vi "JAUS Control Loop.vi"   [LabVIEW 2009]
uses:
  TypeDefs/State Machine/Main State.ctl
  <vilib>/Platform/TimedLoop/XDataNode/XDataNode.xnode
  <vilib>/Platform/TimedLoop/XDataNode/loadlvalarms.vi
  <vilib>/Platform/TimedLoop/XDataNode/timing_clust.ctl
  <vilib>/Platform/TimedLoop/XDataNode/nitl_modes.ctl
  <vilib>/Platform/TimedLoop/XDataNode/wakeup.ctl
  Functional Global Variables/Actions for FG's.ctl
  TypeDefs/Queue TypeDefs/Motor Instruction.ctl
  TypeDefs/Queue TypeDefs/Motor State.ctl
  Remote Control/Motor Command.ctl
  <vilib>/userDefined/High Color/nirio_resource_hc.ctl
  <vilib>/rvi/interface/nirviOpenFPGA/nirviOpenFPGA.xnode
  FPGA Bitfiles/Q_IGVC_2010.lvproj_FPGA Target_FPGA_MAIN.vi.lvbitx
  <vilib>/FPGAPlugInAG/cRIO-9113/nirviIntfOpen_cRIO-9113.vi
  <vilib>/Platform/TimedLoop/XDataNode/XDNodeRunTimeDep.lvlib
  <vilib>/NI_Real-Time Target Support.lvlib
  TypeDefs/Sensor TypeDefs/FPGA Main ref.ctl
types:
  T1 = typedef "Main State.ctl" = enum16{"Startup", "Wait for Init", "Initialize Sensors", "Wait for Saftey Disable", "Check Saftey", "Wait for GO", "Run", "Remote Control", "Stop"}
  T2 = typedef "XDNodeRunTimeDep.lvlib/timing_clust.ctl" = cluster{"Expected End [f-1]":u64, "Actual End [f-1]":u64, "Finished Late? [f-1]":bool, "Expected End [i-1]":u64, "Actual End [i-1]":u64, "Finished Late? [i-1]":bool, "Expected Start [i]":u64, "Actual Start [i]":u64, "Expected Start [f]":u64, "Actual Start [f]":u64, "Source Name":string, "Structure Name":string, "Period":i64, "Deadline":i64, "Offset":i64, "Start":i64, "Priority":i32, "Timeout":i32, "Mode":T3, "Wakeup Reason":T4, "Error":errorcluster, "Source Type":string, "Secondary Source Type":string, "Global End Time":u64, "Global Start Time":u64, "Frame Duration":u64, "Iteration Duration":u64, "Assigned CPU":i32, "I/O Scan Engine Mode":u32}
  T3 = typedef "XDNodeRunTimeDep.lvlib/nitl_modes.ctl" = enum32{"No Change", "Process missed periods, maintain original phase", "Discard missed periods, maintain original phase", "Process missed periods, ignore original phase", "Discard missed periods, ignore original phase"}
  T4 = typedef "XDNodeRunTimeDep.lvlib/wakeup.ctl" = enum32{"Normal", "Aborted", "Asynchronous wakeup", "Timing source error", "Timed loop error", "Timeout"}
  T5 = typedef "Actions for FG's.ctl" = enum16{"Read", "Write"}
  T6 = typedef "nirio_resource_hc.ctl" = tag
  T7 = cluster{"signature":u8[], "vi signatures match":bool, "signature register address":u32, "reset register address":u32, "control register address":u32, "interrupt base address":u32, "Bitstream Version":u32, "DMA Configuration":cluster{"Name":string, "Depth":u32, "Write? (Deprecated:Use Implementation)":bool, "Physical Channel":u32, "Base Address":u32, "Data Width":u32, "Data Type":enum32{"Boolean", "I8", "I16", "I32", "I64", "U8", "U16", "U32", "U64", "FXP"}, "FXP Properties":variant, "Write Window Address":u32, "Implementation":enum16{"niFpgaTargetToHost", "niFpgaHostToTarget", "niFpgaPeerToPeerWriter", "niFpgaPeerToPeerReader", "niCoreTargetToHost", "niCoreHostToTarget"}, "Control Set":u32}[], "run when loaded?":bool, "reset register size in bits":u32, "compilation results xml":string}
  T8 = typedef "Motor State.ctl" = enum16{"Wait", "Initialize", "Check FET", "Run", "Stop"}
  T9 = typedef "Motor Instruction.ctl" = cluster{"Motor State":T8, "Motor Command":T10}
  T10 = typedef "Motor Command.ctl" = cluster{"Speed":i16, "Turn":i16}
  T11 = typedef "FPGA Main ref.ctl" = refnum<k20>
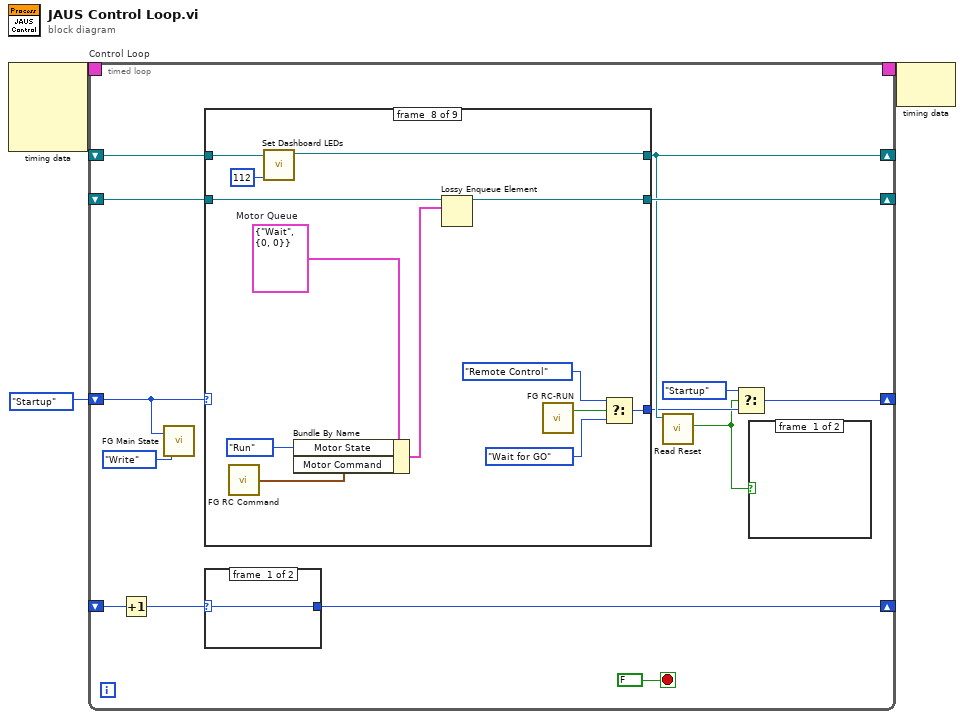
[diagram p0: block diagram]
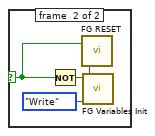
[diagram p2: hidden frame]
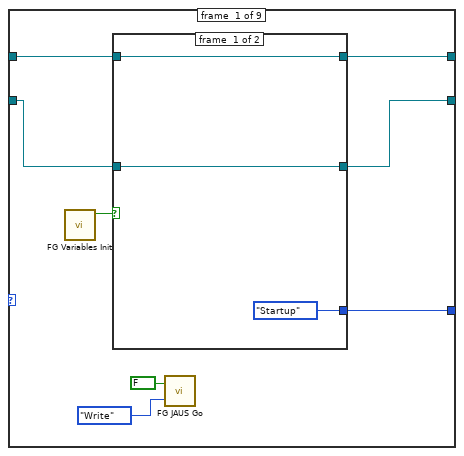
[diagram p3: hidden frame]
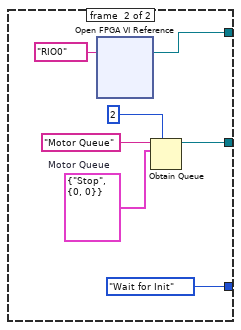
[diagram p4: hidden frame]
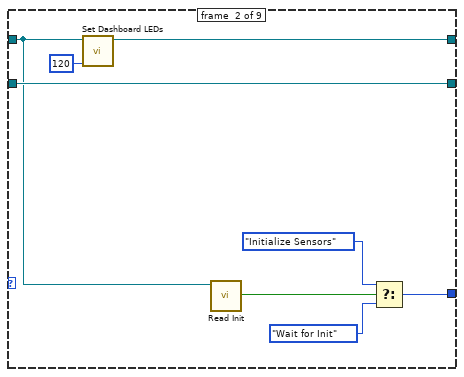
[diagram p5: hidden frame]
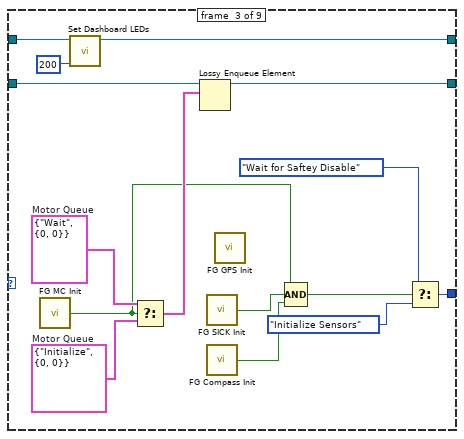
[diagram p6: hidden frame]
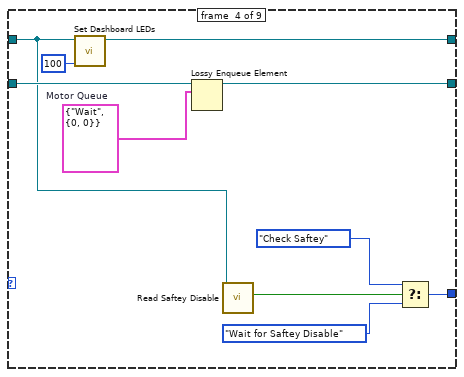
[diagram p7: hidden frame]
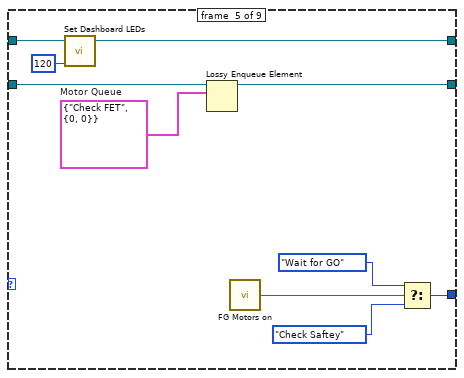
[diagram p8: hidden frame]
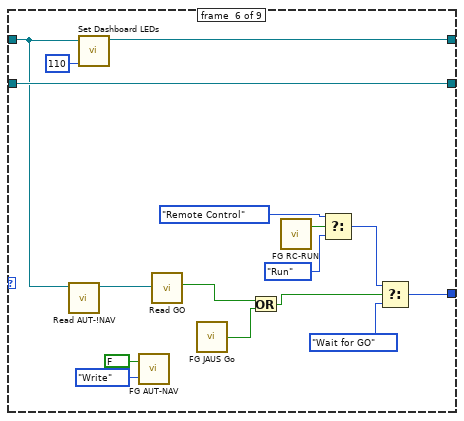
[diagram p9: hidden frame]
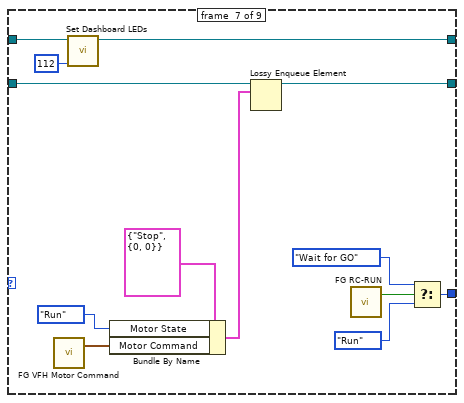
[diagram p10: hidden frame]
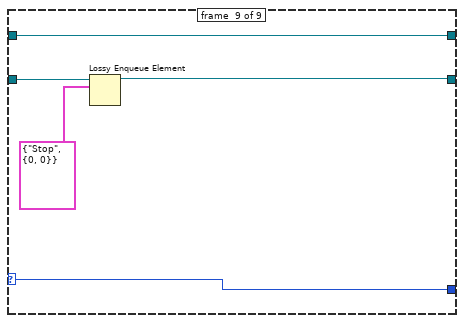
[diagram p11: hidden frame]
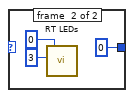
[diagram p12: hidden frame]
diagram:
  n1 = node-c288() -> (w3:T2)  [unwired: 4 in]
  n2 = timed-loop "Control Loop" {
    timing: w3 -> [_]
    timing-out: [_] -> w2
    shift-right: [w14] -> _
    shift-left: _ -> [w16]
    shift-right: [w7] -> _
    shift-left: Main_State."Startup" ("Main State") -> [w11]
    shift-right: [w9] -> _
    shift-left: _ -> [w12]
    shift-right: [w8] -> _
    shift-left: _ -> [w13]
    stop <- FALSE stop-if-true
    n3 = Increment(x=w16) -> (x+1=w15:i32)
    n4 = call "FG Main State.vi"("FG Action"=Actions_for_FG's."Write", "Main State in"=w11) -> ()  [unwired: 1 out]
    n5 = case shown="\"Remote Control\"" w11 {
      selector: w11 -> [_ _ _ _ _ _ _ _ w136]
      tunnel: w13 -> [w23 w51 w59 w74 w84 w98 w110 w127 w135]
      tunnel: w12 -> [w25 w52 w72 w82 w91 w99 w116 w134 w139]
      tunnel: [w24 w53 w65 w76 w86 w102 w112 w128 w136] -> w6
      tunnel: [w27 w52 w60 w75 w85 w99 w111 w123 w137] -> w9
      tunnel: [w26 w50 w58 w73 w83 w97 w109 w122 w135] -> w8
      frame #0 {
        n6 = call "FG Variables Init.vi"() -> ("Variables Init out"=w28:bool)  [unwired: 11 in]
        n7 = case shown="True" w28 {
          tunnel: [w29 w37] -> w26
          tunnel: [w31 w33] -> w27
          tunnel: w25 -> [w31 _]
          tunnel: [Main_State."Startup" ("Main State") Main_State."Wait for Init" ("Main State")] -> w24
          tunnel: w23 -> [w29 _]
          frame #0 {
          }
          frame #1 {
            w35 = T9 {"Motor State"=enum."Stop", "Motor Command"={"Speed"=0, "Turn"=0}}  # Motor Queue
            n8 = xnode "Open FPGA VI Reference"("resource name"=T6 "RIO0") -> ("FPGA VI Reference Out"=w37:T11)  [unwired: 1 in, 1 out]
            n9 = Obtain Queue(max queue size (-1, unlimited)=2, name (unnamed)="Motor Queue", element data type=w35) -> (queue out=w33:refnum<queue>)  [unwired: 2 in, 2 out]
          }
        }
        n10 = call "FG JAUS Go.vi"("FG Action (Read)"=Actions_for_FG's."Write", "Go In"=FALSE) -> ()  [unwired: 1 out]
      }
      frame #1 {
        n11 = call "Set Dashboard LEDs.vi"("Display code"=u8 120, "FPGA VI Reference in"=w51) -> ("FPGA VI Reference out"=w50:T11)  [unwired: 9 in]
        n12 = call "Read Init.vi"("FPGA VI Reference in"=w51) -> ("Init switch"=w57:bool)  [unwired: 7 in, 2 out]
        n13 = Select(t=Main_State."Initialize Sensors" ("Main State out"), s=w57, f=Main_State."Wait for Init" ("Main State out")) -> (s? t:f=w53:T1)
      }
      frame #2 {
        w63 = T9 {"Motor State"=enum."Initialize", "Motor Command"={"Speed"=0, "Turn"=0}}  # Motor Queue
        w64 = T9 {"Motor State"=enum."Wait", "Motor Command"={"Speed"=0, "Turn"=0}}  # Motor Queue
        n14 = call "FG MC Init.vi"() -> ("MC Init out"=w61:bool)  [unwired: 2 in]
        n15 = call "Set Dashboard LEDs.vi"("Display code"=u8 200, "FPGA VI Reference in"=w59) -> ("FPGA VI Reference out"=w58:T11)  [unwired: 9 in]
        n16 = Select(t=w64, s=w61, f=w63) -> (s? t:f=w62:T9)
        n17 = Lossy Enqueue Element(queue=w72, element=w62) -> (queue out=w60:refnum<queue>)  [unwired: 1 in, 3 out]
        n18 = call "FG SICK Init.vi"() -> ("SICK Init out"=w71:bool)  [unwired: 2 in]
        n19 = call "FG Compass Init.vi"() -> ("Compass Init out"=w70:bool)  [unwired: 2 in]
        n20 = call "FG GPS Init.vi"() -> ()  [unwired: 2 in, 1 out]
        n21 = Compound Arithmetic op=AND(w61, w71, w70) -> (w69:bool)
        n22 = Select(t=Main_State."Wait for Saftey Disable" ("Main State out"), s=w69, f=Main_State."Initialize Sensors" ("Main State out")) -> (s? t:f=w65:T1)
      }
      frame #3 {
        w81 = T9 {"Motor State"=enum."Wait", "Motor Command"={"Speed"=0, "Turn"=0}}  # Motor Queue
        n23 = call "Set Dashboard LEDs.vi"("Display code"=u8 100, "FPGA VI Reference in"=w74) -> ("FPGA VI Reference out"=w73:T11)  [unwired: 9 in]
        n24 = Lossy Enqueue Element(queue=w82, element=w81) -> (queue out=w75:refnum<queue>)  [unwired: 1 in, 3 out]
        n25 = call "Read Saftey Disable.vi"("FPGA VI Reference in"=w74) -> ("GO"=w77:bool)  [unwired: 7 in, 2 out]
        n26 = Select(t=Main_State."Check Saftey" ("Main State out"), s=w77, f=Main_State."Wait for Saftey Disable" ("Main State out")) -> (s? t:f=w76:T1)
      }
      frame #4 {
        w92 = T9 {"Motor State"=enum."Check FET", "Motor Command"={"Speed"=0, "Turn"=0}}  # Motor Queue
        n27 = call "Set Dashboard LEDs.vi"("Display code"=u8 120, "FPGA VI Reference in"=w84) -> ("FPGA VI Reference out"=w83:T11)  [unwired: 9 in]
        n28 = Lossy Enqueue Element(queue=w91, element=w92) -> (queue out=w85:refnum<queue>)  [unwired: 1 in, 3 out]
        n29 = call "FG Motors on.vi"() -> ("Motors on ? out"=w88:bool)  [unwired: 2 in]
        n30 = Select(t=Main_State."Wait for GO" ("Main State out"), s=w88, f=Main_State."Check Saftey" ("Main State out")) -> (s? t:f=w86:T1)
      }
      frame #5 {
        n31 = call "Read AUT-!NAV.vi"("FPGA VI Reference in"=w98) -> ("FPGA VI Reference out"=w100:T11)  [unwired: 7 in, 2 out]
        n32 = call "Set Dashboard LEDs.vi"("Display code"=u8 110, "FPGA VI Reference in"=w98) -> ("FPGA VI Reference out"=w97:T11)  [unwired: 9 in]
        n33 = call "FG AUT-NAV.vi"("FG Action (Read)"=Actions_for_FG's."Write", "Aut/!Nav in"=FALSE) -> ()  [unwired: 1 out]
        n34 = call "Read GO.vi"("FPGA VI Reference in"=w100) -> ("GO"=w96:bool)  [unwired: 7 in, 2 out]
        n35 = call "FG JAUS Go.vi"() -> ("Go Out"=w94:bool)  [unwired: 2 in]
        n36 = Or(x=w96, y=w94) -> (x .or. y?=w95:bool)
        n37 = call "FG RC-RUN.vi"() -> ("RC/!Run out"=w106:bool)  [unwired: 3 in]
        n38 = Select(t=Main_State."Remote Control" ("Main State"), s=w106, f=Main_State."Run" ("Main State")) -> (s? t:f=w104:T1)
        n39 = Select(t=w104, s=w95, f=Main_State."Wait for GO" ("Main State")) -> (s? t:f=w102:T1)
      }
      frame #6 {
        n40 = call "FG VFH Motor Command.vi"() -> ("Motor Command out"=w118:T10)  [unwired: 3 in]
        n41 = call "Set Dashboard LEDs.vi"("Display code"=u8 112, "FPGA VI Reference in"=w110) -> ("FPGA VI Reference out"=w109:T11)  [unwired: 9 in]
        n42 = Bundle By Name(cluster=T9 {"Motor State"=enum."Stop", "Motor Command"={"Speed"=0, "Turn"=0}} ("element"), "Motor State"=Motor_State."Run", "Motor Command"=w118) -> (w117:T9)
        n43 = Lossy Enqueue Element(queue=w116, element=w117) -> (queue out=w111:refnum<queue>)  [unwired: 1 in, 3 out]
        n44 = call "FG RC-RUN.vi"() -> ("RC/!Run out"=w113:bool)  [unwired: 3 in]
        n45 = Select(t=Main_State."Wait for GO" ("Main State"), s=w113, f=Main_State."Run" ("Main State")) -> (s? t:f=w112:T1)
      }
      frame #7 {
        w133 = T9 {"Motor State"=enum."Wait", "Motor Command"={"Speed"=0, "Turn"=0}}  # Motor Queue
        n46 = call "FG RC Command.vi"() -> ("Motor Command out"=w125:T10)  [unwired: 2 in]
        n47 = call "Set Dashboard LEDs.vi"("Display code"=u8 112, "FPGA VI Reference in"=w127) -> ("FPGA VI Reference out"=w122:T11)  [unwired: 9 in]
        n48 = Bundle By Name(cluster=w133, "Motor State"=Motor_State."Run", "Motor Command"=w125) -> (w124:T9)
        n49 = Lossy Enqueue Element(queue=w134, element=w124) -> (queue out=w123:refnum<queue>)  [unwired: 1 in, 3 out]
        n50 = call "FG RC-RUN.vi"() -> ("RC/!Run out"=w130:bool)  [unwired: 3 in]
        n51 = Select(t=Main_State."Remote Control" ("Main State"), s=w130, f=Main_State."Wait for GO" ("Main State")) -> (s? t:f=w128:T1)
      }
      frame #8 {
        n52 = Lossy Enqueue Element(queue=w139, element=T9 {"Motor State"=enum."Stop", "Motor Command"={"Speed"=0, "Turn"=0}}) -> (queue out=w137:refnum<queue>)  [unwired: 1 in, 3 out]
      }
    }
    n53 = case shown="Default" w15 {
      selector: w15 -> [w140 _]
      tunnel: [w140 0] -> w14
      frame #0 {
      }
      frame #1 {
        n54 = call <vilib>:"RT LEDs.vi"("State"=3, "LED Num"=0) -> ()  [unwired: 4 in, 2 out]
      }
    }
    n55 = call "Read Reset.vi"("FPGA VI Reference in"=w8) -> ("Reset"=w4:bool)  [unwired: 8 in, 2 out]
    n56 = Select(t=Main_State."Startup", s=w4, f=w6) -> (s? t:f=w7:T1)
    n57 = case shown="True" w4 {
      selector: w4 -> [_ w18]
      frame #0 {
      }
      frame #1 {
        w19 = Actions_for_FG's."Write" ("FG Action (Read)")
        n58 = Not(x=w18) -> (.not. x?=w20:bool)
        n59 = call "FG RESET.vi"("FG Action (Read)"=w19, "RESET in"=w18) -> ()  [unwired: 1 out]
        n60 = call "FG Variables Init.vi"("FG Action"=w19, "Variables Init in"=w20) -> ()  [unwired: 9 in, 1 out]
      }
    }
  }
  n61 = node-c288(w2) -> ()  [unwired: 1 out]
